vi "Example.vi"() -> ()   [LabVIEW 2021]
doc: "Example showing basic usage of the BR_error_handling library. \nTo be able to use this library, it is necessary to initialize error handler first (Init Error Handler.vi), which will search for the XML file in format: '*-errors.txt' with specified custom errors in application directory and its subfolders. \nTo generate custom error, which format is specified in TXT file, use Generate Error.vi and wire required error code to the input with eventual inputs for error description.\nCase structure easily shows multiple use-cases and situations that can occure during using this library."
panel:
  out "Generated Error 9":errorcluster
  out "Generated Error 4":errorcluster
  out "Generated Error 2":errorcluster
  out "Generated Error 1":errorcluster
  out "Generated Error 8":errorcluster
  out "Generated Error 7":errorcluster
  out "Generated Error 6":errorcluster
  out "Generated Error 3":errorcluster
  out "Generated Error 5":errorcluster
  # "Overview: Demonstrates how the error_handling library works, and how to wire inputs to Generate Error function. \nInstructions:\n1. Examine the different cases in the block diagram, showing different methods of wiring inputs to error message.\n2. Select the case to be executed from Error format type enum.\n3. Run the VI."
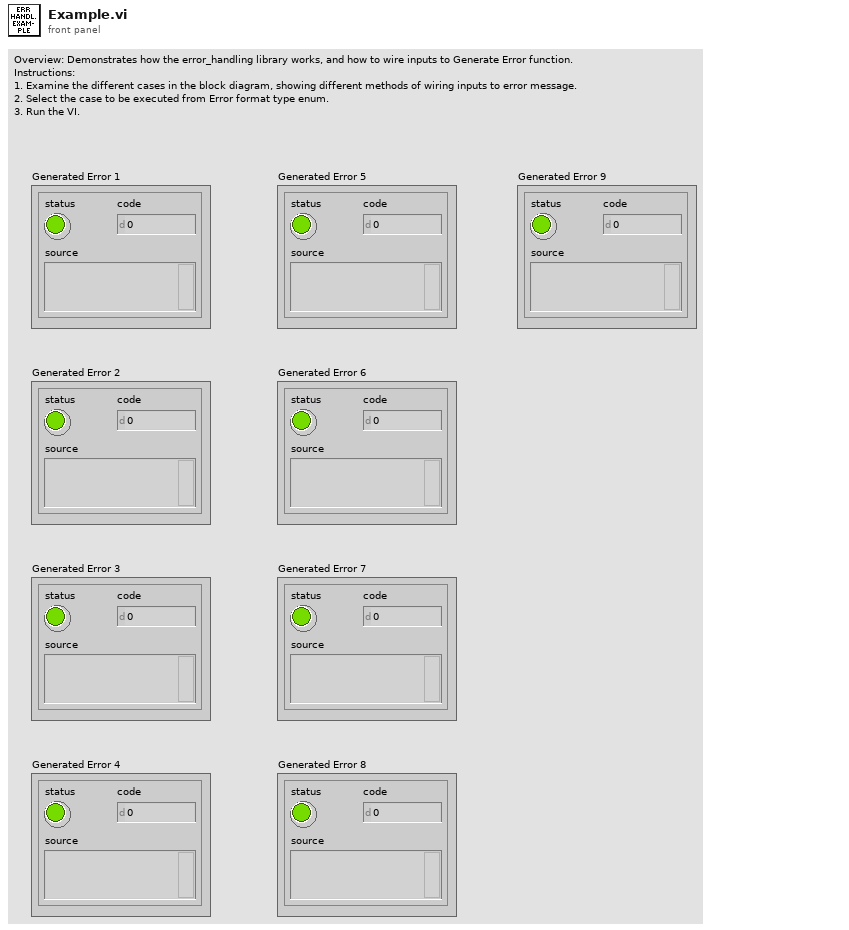
[diagram p1: front panel]
types:
  T1 = cluster{string, "seconds since 1Jan1904":timestamp}
  T2 = cluster{string, i32[], cluster{dbl, bool, bool, i32[]}}
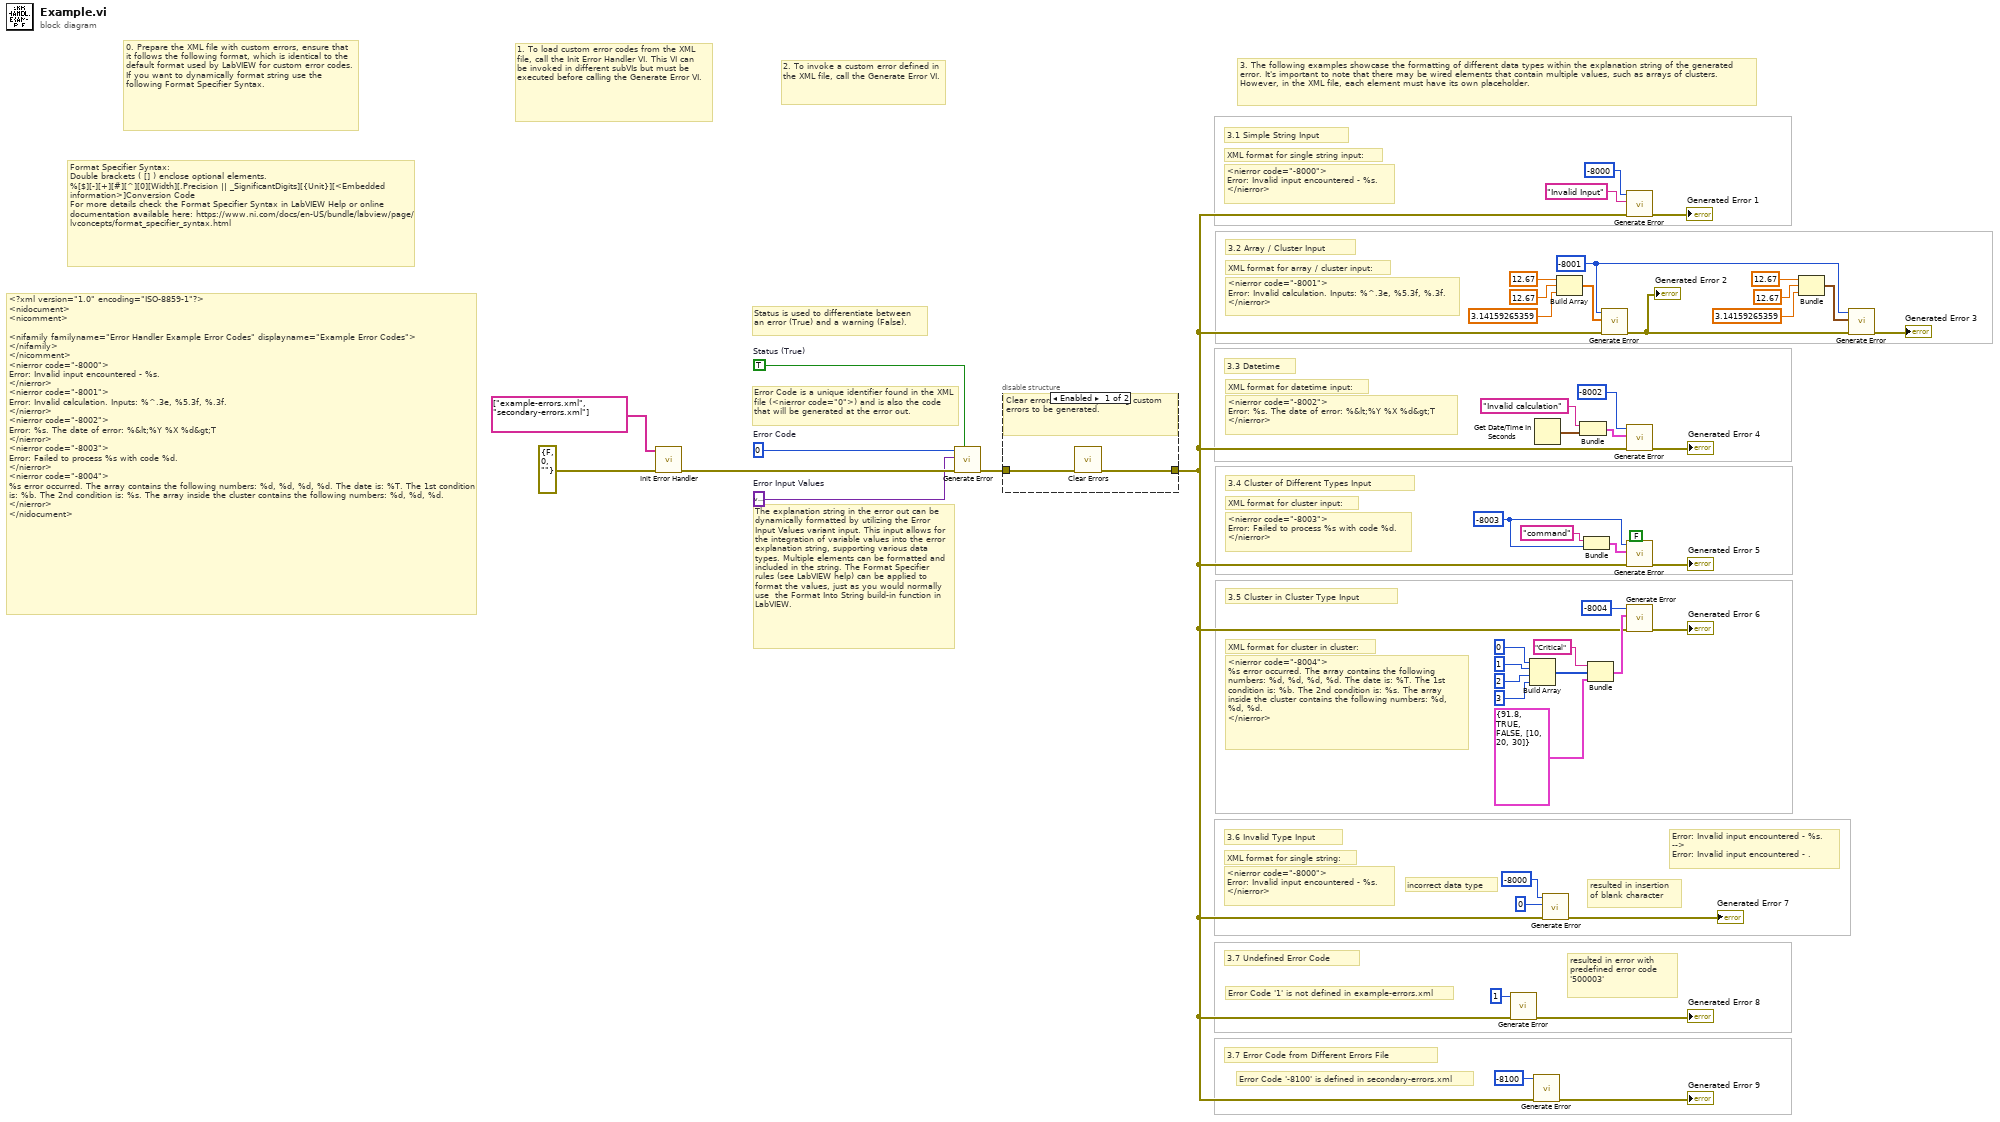
[diagram p0: block diagram]
diagram:
  w22 = variant  # Error Input Values
  w23 = 0  # Error Code
  w24 = TRUE  # Status (True)
  w18 = -8001 ("Error Code")
  w12 = -8003 ("Error Code")
  # "Error Code '-8100' is defined in secondary-errors.xml"
  # "3.7 Error Code from Different Errors File"
  # "Format Specifier Syntax:\nDouble brackets ( [] ) enclose optional elements.\n%[$][-][+][#][^][0][Width][.Precision || _SignificantDigits][{Unit}][<Embedded information>]Conversion Code\nFor more details check the Format Specifier Syntax in LabVIEW Help or online documentation available here: https://www.ni.com/docs/en-US/bundle/labview/page/lvconcepts/format_specifier_syntax.html"
  # "XML format for datetime input:"
  # "<nierror code=\"-8002\">\nError: %s. The date of error: %&lt;%Y %X %d&gt;T\n</nierror>"
  # "3.3 Datetime"
  # "3. The following examples showcase the formatting of different data types within the explanation string of the generated error. It's important to note that there may be wired elements that contain multiple values, such as arrays of clusters. However, in the XML file, each element must have its own placeholder."
  # "The explanation string in the error out can be dynamically formatted by utilizing the Error Input Values variant input. This input allows for the integration of variable values into the error explanation string, supporting various data types. Multiple elements can be formatted and included in the string. The Format Specifier rules (see LabVIEW help) can be applied to format the values, just as you would normally use  the Format Into String build-in function in LabVIEW."
  # "Error Code is a unique identifier found in the XML file (<nierror code=\"0\">) and is also the code that will be generated at the error out."
  # "Status is used to differentiate between an error (True) and a warning (False)."
  # "<?xml version=\"1.0\" encoding=\"ISO-8859-1\"?>\n<nidocument>\n<nicomment>\n\n<nifamily familyname=\"Error Handler Example Error Codes\" displayname=\"Example Error Codes\">\n</nifamily>\n</nicomment>\n<nierror code=\"-8000\">\nError: Invalid input encountered - %s.\n</nierror>\n<nierror code=\"-8001\">\nError: Invalid calculation. Inputs: %^.3e, %5.3f, %.3f.\n</nierror>\n<nierror code=\"-8002\">\nError: %s. The date of error: %&lt;%Y %X %d&gt;T\n</nierror>\n<nierror code=\"-8003\">\nError: Failed to process %s with code %d.\n</nierror>\n<nierror code=\"-8004\">\n%s error occurred. The array contains the following numbers: %d, %d, %d, %d. The date is: %T. The 1st condition is: %b. The 2nd condition is: %s. The array inside the cluster contains the following numbers: %d, %d, %d.\n</nierror>\n</nidocument>"
  # "0. Prepare the XML file with custom errors, ensure that it follows the following format, which is identical to the default format used by LabVIEW for custom error codes. \nIf you want to dynamically format string use the following Format Specifier Syntax."
  # "2. To invoke a custom error defined in the XML file, call the Generate Error VI."
  # "1. To load custom error codes from the XML file, call the Init Error Handler VI. This VI can be invoked in different subVIs but must be executed before calling the Generate Error VI."
  # "resulted in error with predefined error code '500003'"
  # "Error Code '1' is not defined in example-errors.xml"
  # "3.7 Undefined Error Code"
  # "Error: Invalid input encountered - %s.\n-->\nError: Invalid input encountered - ."
  # "resulted in insertion of blank character"
  # "incorrect data type"
  # "XML format for single string:"
  # "<nierror code=\"-8000\">\nError: Invalid input encountered - %s.\n</nierror>"
  # "3.6 Invalid Type Input"
  # "XML format for cluster in cluster:"
  # "<nierror code=\"-8004\">\n%s error occurred. The array contains the following numbers: %d, %d, %d, %d. The date is: %T. The 1st condition is: %b. The 2nd condition is: %s. The array inside the cluster contains the following numbers: %d, %d, %d.\n</nierror>"
  # "3.5 Cluster in Cluster Type Input"
  # "XML format for array / cluster input:"
  # "<nierror code=\"-8001\">\nError: Invalid calculation. Inputs: %^.3e, %5.3f, %.3f.\n</nierror>"
  # "3.2 Array / Cluster Input"
  # "XML format for cluster input:"
  # "<nierror code=\"-8003\">\nError: Failed to process %s with code %d.\n</nierror>"
  # "3.4 Cluster of Different Types Input"
  # "XML format for single string input:"
  # "<nierror code=\"-8000\">\nError: Invalid input encountered - %s.\n</nierror>"
  # "3.1 Simple String Input"
  n1 = call "Init Error Handler.vi"("error in"=errorcluster {"status"=FALSE, "code"=0, "source"=""}, "File Names (Optional)"=string[] ["example-errors.xml", "secondary-errors.xml"]) -> ("error out"=w25:errorcluster)  [unwired: 9 in]
  n2 = call "Generate Error.vi"("Status (True)"=w24, "error in"=w25, "Error Input Values"=w22, "Error Code"=w23) -> ("Generated Error"=w13:errorcluster)  [unwired: 7 in]
  n3 = disable-structure shown="Enabled" {
    disable-tunnel: w13 -> [w51 w52]
    disable-tunnel: [w50 w52] -> w1
    frame Enabled {
      # "Clear errors to allow upcoming custom errors to be generated."
      n4 = call <vilib>:"Clear Errors.vi"("error in (no error)"=w51) -> ("error out"=w50:errorcluster)  [unwired: 5 in, 1 out]
    }
    frame Disabled {
      # "Do not clear the generated error"
    }
  }
  n5 = call "Generate Error.vi"("error in"=w1, "Error Code"=1) -> ("Generated Error"=→"Generated Error 8":errorcluster)  [unwired: 9 in]
  n6 = Build Array(0, 1, 2, 3) -> (w42:i32[])
  n7 = call "Generate Error.vi"("error in"=w1, "Error Code"=-8100) -> ("Generated Error"=→"Generated Error 9":errorcluster)  [unwired: 9 in]
  n8 = Get Date/Time In Seconds() -> (seconds since 1Jan1904=w8:timestamp)
  n9 = call "Generate Error.vi"("error in"=w1, "Error Input Values"=0, "Error Code"=-8000) -> ("Generated Error"=→"Generated Error 7":errorcluster)  [unwired: 8 in]
  n10 = Build Array(12.67, 12.67, 3.14159265359) -> (w46:dbl[])
  n11 = Bundle("Invalid calculation", "seconds since 1Jan1904"=w8) -> (w6:T1)  [unwired: 1 in]
  n12 = Bundle("command", "Error Code"=w12) -> (w47:cluster{string, "Error Code":i32})  [unwired: 1 in]
  n13 = Bundle("Critical", w42, cluster{dbl, bool, bool, i32[]} {91.8, TRUE, FALSE, [10, 20, 30]}) -> (w41:T2)  [unwired: 1 in]
  n14 = call "Generate Error.vi"("error in"=w1, "Error Input Values"=w46, "Error Code"=w18) -> ("Generated Error"=w19:errorcluster)  [unwired: 8 in]
  "Generated Error 2" <- w19
  n15 = call "Generate Error.vi"("error in"=w1, "Error Input Values"="Invalid Input", "Error Code"=-8000) -> ("Generated Error"=→"Generated Error 1":errorcluster)  [unwired: 8 in]
  n16 = call "Generate Error.vi"("error in"=w1, "Error Input Values"=w6, "Error Code"=-8002) -> ("Generated Error"=→"Generated Error 4":errorcluster)  [unwired: 8 in]
  n17 = call "Generate Error.vi"("Status (True)"=FALSE, "error in"=w1, "Error Input Values"=w47, "Error Code"=w12) -> ("Generated Error"=→"Generated Error 5":errorcluster)  [unwired: 7 in]
  n18 = call "Generate Error.vi"("error in"=w1, "Error Input Values"=w41, "Error Code"=-8004) -> ("Generated Error"=→"Generated Error 6":errorcluster)  [unwired: 8 in]
  n19 = Bundle(12.67, 12.67, 3.14159265359) -> (w14:cluster{dbl, dbl, dbl})  [unwired: 1 in]
  n20 = call "Generate Error.vi"("error in"=w19, "Error Input Values"=w14, "Error Code"=w18) -> ("Generated Error"=→"Generated Error 3":errorcluster)  [unwired: 8 in]
